vi "RegisterMap_RegMap Mask.vi"(8 "LSB":u16, 9 "MSB":u16) -> (1 "Mask":u16 format="%04x")   [LabVIEW 2010]
doc: "This VI generates the bit mask for the element in the register based on the MSB and LSB positions. The mask will be of the form 0x0000100, where the 1s represent the desired bits in the register.\n\nInputs:\nMSB - (u16) position of the MSB of the item\nLSB - (u16) position of the LSB of the item\n\nOutput:\nMask - (u16) register mask to apply for the input item"
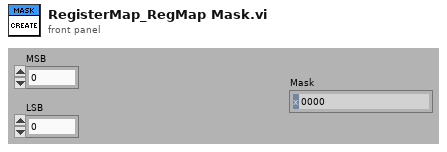
[diagram p1: front panel]
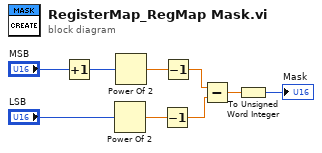
[diagram p0: block diagram]
diagram:
  n1 = Increment(x="MSB") -> (x+1=w8:u16)
  n2 = Power Of 2(x="LSB") -> (2^x=w6:dbl)
  n3 = Power Of 2(x=w8) -> (2^x=w7:dbl)
  n4 = Decrement(x=w6) -> (x-1=w4:dbl)
  n5 = Decrement(x=w7) -> (x-1=w5:dbl)
  n6 = Subtract(x=w5, y=w4) -> (x-y=w3:dbl)
  n7 = To Unsigned Word Integer(number=w3) -> (unsigned 16bit integer=→"Mask":u16)
